vi "CFTS-Defaults File Path.vi"() -> (0 "Path":path)   [LabVIEW 2020]
uses:
  <vilib>/Utility/sysdir.llb/System Directory Type.ctl
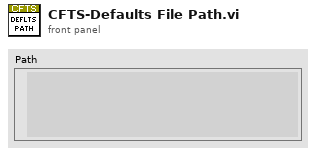
[diagram p1: front panel]
types:
  T1 = typedef "System Directory Type.ctl" = i32
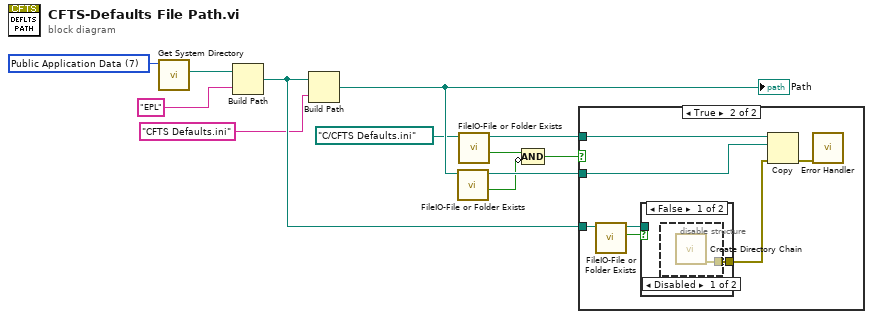
[diagram p0: block diagram]
diagram:
  w12 = T1 7 items=["User Home"=0, "User Desktop"=1, "User Documents"=2, "User Application Data"=3, "User Preferences"=4, "User Temporary"=5, "Public Documents"=6, "Public Application Data"=7, "Public Preferences"=8, "Public Cache"=13, "System Core Libraries"=9, "System Installed Libraries"=10, "Application Files"=11, "Boot Volume Root"=12] ("system directory type")
  n1 = call <vilib>:"Get System Directory.vi"("system directory type"=w12) -> ("system directory"=w11:path)  [unwired: 10 in]
  n2 = Build Path(base path=w11, name or relative path="EPL") -> (appended path=w9:path)
  n3 = Build Path(base path=w9, name or relative path="CFTS Defaults.ini") -> (appended path=w7:path)
  "Path" <- w7
  n4 = call "FileIO-File or Folder Exists.vi"("path"=w7) -> ("Exists?"=w3:bool, "dup path"=w6:path)  [unwired: 7 in, 2 out]
  n5 = call "FileIO-File or Folder Exists.vi"("path"=path "C:/CFTS Defaults.ini" ("configuration file path")) -> ("Exists?"=w4:bool, "dup path"=w1:path)  [unwired: 7 in, 2 out]
  n6 = Compound Arithmetic op=AND(w4, invert w3) -> (w2:bool)
  n7 = case shown="True" w2 {
    tunnel: w9 -> [_ w19]
    tunnel: w6 -> [_ w16]
    tunnel: w1 -> [_ w14]
    frame False {
    }
    frame True {
      n8 = call "FileIO-File or Folder Exists.vi"("path"=w19) -> ("Directory?"=w18:bool, "dup path"=w17:path)  [unwired: 7 in, 2 out]
      n9 = case shown="False" w18 {
        tunnel: w17 -> [_ _]
        tunnel: [w20 _] -> w13
        frame False {
          n10 = disable-structure shown="Disabled" {
            disable-tunnel: [w21 _] -> w20
            frame Disabled {
              n11 = call "Create Directory Chain.vi"() -> ("Error Out"=w21:errorcluster)  [unwired: 10 in, 1 out]
            }
            frame Enabled {
            }
          }
        }
        frame True {
        }
      }
      n12 = Copy(8:w13, 10:w16, 11:w14) -> (0:w15:errorcluster)  [unwired: 2 in, 2 out]
      n13 = call "Error Handler.vi"("error in (no error)"=w15) -> ()  [unwired: 13 in, 2 out]
    }
  }
